vi "nanocal -- nuclear schottky fit V3.vi"() -> ()   [LabVIEW 2020] (continued)
\"κ0\"-> 0.000000001075  , \"mm1\"-> 0.000000000000  , \"mm2\"-> 0.000000000000  , \"mm3\"-> 0.000000000000  , \"T\"->  0.197000000000  , \"B\"-> 8.000000000000  , \"θ\"-> 90.000000000000  |>   , \r4103 ->   <| \"ζ\"->  0.162645417184  , \"τ1\"-> 0.023693851446  , \"τS\"-> 0.062400062170  , \"τN\"-> 0.026326088223  , \"τC\"-> 0.001322053294  , \"κ0\"-> 0.000000001070  , \"mm1\"-> 0.000000000000  , \"mm2\"-> 0.000000000000  , \"mm3\"-> 0.000000000000  , \"T\"->  0.197000000000  , \"B\"-> 7.000000000000  , \"θ\"-> 90.000000000000  |>   , \r4104 ->   <| \"ζ\"->  0.149904026692  , \"τ1\"-> 0.020347243982  , \"τS\"-> 0.075273674904  , \"τN\"-> 0.020640082408  , \"τC\"-> 0.001432916876  , \"κ0\"-> 0.000000001050  , \"mm1\"-> 0.000000000000  , \"mm2\"-> 0.000000000000  , \"mm3\"-> 0.000000000000  , \"T\"->  0.197000000000  , \"B\"-> 5.000000000000  , \"θ\"-> 90.000000000000  |>   , \r4105 ->   <| \"ζ\"->  0.121305227705  , \"τ1\"-> 0.032098202143  , \"τS\"-> 0.011865067519  , \"τN\"-> 0.005878702730  , \"τC\"-> 0.002147559783  , \"κ0\"-> 0.000000001032  , \"mm1\"-> 0.000000000000  , \"mm2\"-> 0.000000000000  , \"mm3\"-> 0.000000000000  , \"T\"->  0.197000000000  , \"B\"-> 0.000000000000  , \"θ\"-> 90.000000000000  |>   , \r4106 ->   <| \"ζ\"->  0.000000000000  , \"τ1\"-> 0.000000000000  , \"τS\"-> 0.000000000000  , \"τN\"-> 0.000000000000  , \"τC\"-> 0.000000000000  , \"κ0\"-> 0.000000000000  , \"mm1\"-> 0.000000000000  , \"mm2\"-> 0.000000000000  , \"mm3\"-> 0.000000000000  , \"T\"->  1.550000000000  , \"B\"-> 0.000000000000  , \"θ\"-> 90.000000000000  |>   , \r4107 ->   <| \"ζ\"->  0.000000000000  , \"τ1\"-> 0.000000000000  , \"τS\"-> 0.000000000000  , \"τN\"-> 0.000000000000  , \"τC\"-> 0.000000000000  , \"κ0\"-> 0.000000000000  , \"mm1\"-> 0.000000000000  , \"mm2\"-> 0.000000000000  , \"mm3\"-> 0.000000000000  , \"T\"->  1.000000000000  , \"B\"-> 0.000000000000  , \"θ\"-> 90.000000000000  |>   , \r4108 ->   <| \"ζ\"->  0.000000000000  , \"τ1\"-> 0.000000000000  , \"τS\"-> 0.000000000000  , \"τN\"-> 0.000000000000  , \"τC\"-> 0.000000000000  , \"κ0\"-> 0.000000000000  , \"mm1\"-> 0.000000000000  , \"mm2\"-> 0.000000000000  , \"mm3\"-> 0.000000000000  , \"T\"->  0.670000000000  , \"B\"-> 0.000000000000  , \"θ\"-> 90.000000000000  |>   , \r4110 ->   <| \"ζ\"->  0.282256587364  , \"τ1\"-> 0.041594214767  , \"τS\"-> 0.086147539104  , \"τN\"-> 0.179856853536  , \"τC\"-> 0.001095910669  , \"κ0\"-> 0.000000000648  , \"mm1\"-> 0.000000000000  , \"mm2\"-> 0.000000000000  , \"mm3\"-> 0.000000000000  , \"T\"->  0.160000000000  , \"B\"-> 12.000000000000  , \"θ\"-> 30.000000000000  |>   , \r4112 ->   <| \"ζ\"->  0.271363353906  , \"τ1\"-> 0.041443755069  , \"τS\"-> 0.099499603649  , \"τN\"-> 0.147006393002  , \"τC\"-> 0.001049141338  , \"κ0\"-> 0.000000000745  , \"mm1\"-> 0.000000000000  , \"mm2\"-> 0.000000000000  , \"mm3\"-> 0.000000000000  , \"T\"->  0.170000000000  , \"B\"-> 12.000000000000  , \"θ\"-> 30.000000000000  |>   , \r4113 ->   <| \"ζ\"->  0.338385515343  , \"τ1\"-> 0.049005471612  , \"τS\"-> 0.154718584573  , \"τN\"-> 0.405362096342  , \"τC\"-> 0.001218418583  , \"κ0\"-> 0.000000000425  , \"mm1\"-> 0.000000000000  , \"mm2\"-> 0.000000000000  , \"mm3\"-> 0.000000000000  , \"T\"->  0.140000000000  , \"B\"-> 12.000000000000  , \"θ\"-> 30.000000000000  |>   , \r4114 ->   <| \"ζ\"->  0.206936374087  , \"τ1\"-> 0.035561389628  , \"τS\"-> 0.073638069843  , \"τN\"-> 0.086460784567  , \"τC\"-> 0.001118747808  , \"κ0\"-> 0.000000001040  , \"mm1\"-> 0.000000000000  , \"mm2\"-> 0.000000000000  , \"mm3\"-> 0.000000000000  , \"T\"->  0.200000000000  , \"B\"-> 12.000000000000  , \"θ\"-> 30.000000000000  |>   , \r4115 ->   <| \"ζ\"->  0.117063376722  , \"τ1\"-> 0.028106174799  , \"τS\"-> 0.053754257200  , \"τN\"-> 0.028698663234  , \"τC\"-> 0.001316309287  , \"κ0\"-> 0.000000001351  , \"mm1\"-> 0.000000000000  , \"mm2\"-> 0.000000000000  , \"mm3\"-> 0.000000000000  , \"T\"->  0.250000000000  , \"B\"-> 12.000000000000  , \"θ\"-> 30.000000000000  |>   , \r4116 ->   <| \"ζ\"->  0.083503200365  , \"τ1\"-> 0.024154552454  , \"τS\"-> 0.043596505291  , \"τN\"-> 0.014415309061  , \"τC\"-> 0.001558050220  , \"κ0\"-> 0.000000001736  , \"mm1\"-> 0.000000000000  , \"mm2\"-> 0.000000000000  , \"mm3\"-> 0.000000000000  , \"T\"->  0.300000000000  , \"B\"-> 12.000000000000  , \"θ\"-> 30.000000000000  |>   , \r4117 ->   <| \"ζ\"->  0.066204854396  , \"τ1\"-> 0.022115453498  , \"τS\"-> 0.040315193272  , \"τN\"-> 0.009107814509  , \"τC\"-> 0.001932832854  , \"κ0\"-> 0.000000002123  , \"mm1\"-> 0.000000000000  , \"mm2\"-> 0.000000000000  , \"mm3\"-> 0.000000000000  , \"T\"->  0.360000000000  , \"B\"-> 12.000000000000  , \"θ\"-> 30.000000000000  |>   , \r4118 ->   <| \"ζ\"->  0.047151602613  , \"τ1\"-> 0.020449467018  , \"τS\"-> 0.034469980201  , \"τN\"-> 0.004383898226  , \"τC\"-> 0.002055617066  , \"κ0\"-> 0.000000002642  , \"mm1\"-> 0.000000000000  , \"mm2\"-> 0.000000000000  , \"mm3\"-> 0.000000000000  , \"T\"->  0.430000000000  , \"B\"-> 12.000000000000  , \"θ\"-> 30.000000000000  |>   , \r4119 ->   <| \"ζ\"->  0.034119623194  , \"τ1\"-> 0.019653386186  , \"τS\"-> 0.029887540037  , \"τN\"-> 0.002225158248  , \"τC\"-> 0.003041304002  , \"κ0\"-> 0.000000003299  , \"mm1\"-> 0.000000000000  , \"mm2\"-> 0.000000000000  , \"mm3\"-> 0.000000000000  , \"T\"->  0.530000000000  , \"B\"-> 12.000000000000  , \"θ\"-> 30.000000000000  |>   , \r4120 ->   <| \"ζ\"->  0.027646253689  , \"τ1\"-> 0.019846033328  , \"τS\"-> 0.026627790851  , \"τN\"-> 0.001396225568  , \"τC\"-> 0.003492513642  , \"κ0\"-> 0.000000003909  , \"mm1\"-> 0.000000000000  , \"mm2\"-> 0.000000000000  , \"mm3\"-> 0.000000000000  , \"T\"->  0.620000000000  , \"B\"-> 12.000000000000  , \"θ\"-> 30.000000000000  |>   , \r4121 ->   <| \"ζ\"->  0.021289486927  , \"τ1\"-> 0.020280543944  , \"τS\"-> 0.021209329853  , \"τN\"-> 0.000861491542  , \"τC\"-> 0.004079950225  , \"κ0\"-> 0.000000005431  , \"mm1\"-> 0.000000000000  , \"mm2\"-> 0.000000000000  , \"mm3\"-> 0.000000000000  , \"T\"->  0.830000000000  , \"B\"-> 12.000000000000  , \"θ\"-> 30.000000000000  |>   , \r4122 ->   <| \"ζ\"->  0.017438026946  , \"τ1\"-> 0.020462647610  , \"τS\"-> 0.016753258897  , \"τN\"-> 0.000520420479  , \"τC\"-> 0.004207921766  , \"κ0\"-> 0.000000007613  , \"mm1\"-> 0.000000000000  , \"mm2\"-> 0.000000000000  , \"mm3\"-> 0.000000000000  , \"T\"->  1.130000000000  , \"B\"-> 12.000000000000  , \"θ\"-> 30.000000000000  |>   , \r4123 ->   <| \"ζ\"->  0.016024491492  , \"τ1\"-> 0.020653048802  , \"τS\"-> 0.011065599363  , \"τN\"-> 0.000170904127  , \"τC\"-> 0.004501051440  , \"κ0\"-> 0.000000013123  , \"mm1\"-> 0.000000000000  , \"mm2\"-> 0.000000000000  , \"mm3\"-> 0.000000000000  , \"T\"->  1.900000000000  , \"B\"-> 12.000000000000  , \"θ\"-> 30.000000000000  |>   , \r4124 ->   <| \"ζ\"->  0.018571356814  , \"τ1\"-> 0.020537072361  , \"τS\"-> 0.007110096223  , \"τN\"-> 0.000081792866  , \"τC\"-> 0.004406299379  , \"κ0\"-> 0.000000023512  , \"mm1\"-> 0.000000000000  , \"mm2\"-> 0.000000000000  , \"mm3\"-> 0.000000000000  , \"T\"->  3.100000000000  , \"B\"-> 12.000000000000  , \"θ\"-> 30.000000000000  |>   , \r8026 ->   <| \"ζ\"->  0.226997000000  , \"τ1\"-> 0.061001000000  , \"τS\"-> 0.056065000000  , \"τN\"-> 0.451284000000  , \"τC\"-> 0.001917000000  , \"κ0\"-> 0.000000000541  , \"mm1\"-> 0.000000000000  , \"mm2\"-> 0.000000000000  , \"mm3\"-> 0.000000000000  , \"T\"->  0.127000000000  , \"B\"-> 12.000000000000  , \"θ\"-> 60.000000000000  |>   , \r8027 ->   <| \"ζ\"->  0.172926301574  , \"τ1\"-> 0.059570486348  , \"τS\"-> 0.050344582002  , \"τN\"-> 0.265837950917  , \"τC\"-> 0.001945823967  , \"κ0\"-> 0.000000000779  , \"mm1\"-> 0.000000000000  , \"mm2\"-> 0.000000000000  , \"mm3\"-> 0.000000000000  , \"T\"->  0.150000000000  , \"B\"-> 12.000000000000  , \"θ\"-> 60.000000000000  |>   , \r8028 ->   <| \"ζ\"->  0.148902664674  , \"τ1\"-> 0.053249092192  , \"τS\"-> 0.052262765310  , \"τN\"-> 0.169789454991  , \"τC\"-> 0.002259759037  , \"κ0\"-> 0.000000000876  , \"mm1\"-> 0.000000000000  , \"mm2\"-> 0.000000000000  , \"mm3\"-> 0.000000000000  , \"T\"->  0.179000000000  , \"B\"-> 12.000000000000  , \"θ\"-> 60.000000000000  |>   , \r8029 ->   <| \"ζ\"->  0.112487722964  , \"τ1\"-> 0.051395902330  , \"τS\"-> 0.046676654477  , \"τN\"-> 0.101658461283  , \"τC\"-> 0.002724334068  , \"κ0\"-> 0.000000001186  , \"mm1\"-> 0.000000000000  , \"mm2\"-> 0.000000000000  , \"mm3\"-> 0.000000000000  , \"T\"->  0.200000000000  , \"B\"-> 12.000000000000  , \"θ\"-> 60.000000000000  |>   , \r8030 ->   <| \"ζ\"->  0.086003233788  , \"τ1\"-> 0.048496801153  , \"τS\"-> 0.044168635092  , \"τN\"-> 0.056305790348  , \"τC\"-> 0.004231546790  , \"κ0\"-> 0.000000001462  , \"mm1\"-> 0.000000000000  , \"mm2\"-> 0.000000000000  , \"mm3\"-> 0.000000000000  , \"T\"->  0.240000000000  , \"B\"-> 12.000000000000  , \"θ\"-> 60.000000000000  |>   , \r8031 ->   <| \"ζ\"->  0.057384090127  , \"τ1\"-> 0.040985919910  , \"τS\"-> 0.035958032989  , \"τN\"-> 0.030082348419  , \"τC\"-> 0.004188092728  , \"κ0\"-> 0.000000001825  , \"mm1\"-> 0.000000000000  , \"mm2\"-> 0.000000000000  , \"mm3\"-> 0.000000000000  , \"T\"->  0.287000000000  , \"B\"-> 12.000000000000  , \"θ\"-> 60.000000000000  |>   , \r8032 ->   <| \"ζ\"->  0.043350504485  , \"τ1\"-> 0.035291986431  , \"τS\"-> 0.032748907144  , \"τN\"-> 0.017241468603  , \"τC\"-> 0.005241482788  , \"κ0\"-> 0.000000002152  , \"mm1\"-> 0.000000000000  , \"mm2\"-> 0.000000000000  , \"mm3\"-> 0.000000000000  , \"T\"->  0.330000000000  , \"B\"-> 12.000000000000  , \"θ\"-> 60.000000000000  |>   , \r8033 ->   <| \"ζ\"->  0.024739987039  , \"τ1\"-> 0.030389077736  , \"τS\"-> 0.031546934636  , \"τN\"-> 0.007979884290  , \"τC\"-> 0.005340402456  , \"κ0\"-> 0.000000002860  , \"mm1\"-> 0.000000000000  , \"mm2\"-> 0.000000000000  , \"mm3\"-> 0.000000000000  , \"T\"->  0.430000000000  , \"B\"-> 12.000000000000  , \"θ\"-> 60.000000000000  |>   , \r8034 ->   <| \"ζ\"->  0.017670248411  , \"τ1\"-> 0.029826184303  , \"τS\"-> 0.029273717282  , \"τN\"-> 0.004773699195  , \"τC\"-> 0.006202011547  , \"κ0\"-> 0.000000003450  , \"mm1\"-> 0.000000000000  , \"mm2\"-> 0.000000000000  , \"mm3\"-> 0.000000000000  , \"T\"->  0.510000000000  , \"B\"-> 12.000000000000  , \"θ\"-> 60.000000000000  |>   , \r8035 ->   <| \"ζ\"->  0.013857502217  , \"τ1\"-> 0.024739987039  , \"τS\"-> 0.022532031675  , \"τN\"-> 0.002673871537  , \"τC\"-> 0.006319058754  , \"κ0\"-> 0.000000004207  , \"mm1\"-> 0.000000000000  , \"mm2\"-> 0.000000000000  , \"mm3\"-> 0.000000000000  , \"T\"->  0.620000000000  , \"B\"-> 12.000000000000  , \"θ\"-> 60.000000000000  |>   , \r8036 ->   <| \"ζ\"->  0.008522550050  , \"τ1\"-> 0.024739987039  , \"τS\"-> 0.016706411949  , \"τN\"-> 0.001416010776  , \"τC\"-> 0.006938274982  , \"κ0\"-> 0.000000005839  , \"mm1\"-> 0.000000000000  , \"mm2\"-> 0.000000000000  , \"mm3\"-> 0.000000000000  , \"T\"->  0.830000000000  , \"B\"-> 12.000000000000  , \"θ\"-> 60.000000000000  |>   , \r8037 ->   <| \"ζ\"->  0.005755105359  , \"τ1\"-> 0.019922509440  , \"τS\"-> 0.014656977648  , \"τN\"-> 0.000670306824  , \"τC\"-> 0.007908429886  , \"κ0\"-> 0.000000008190  , \"mm1\"-> 0.000000000000  , \"mm2\"-> 0.000000000000  , \"mm3\"-> 0.000000000000  , \"T\"->  1.130000000000  , \"B\"-> 12.000000000000  , \"θ\"-> 60.000000000000  |>   , \r8038 ->   <| \"ζ\"->  0.003814320430  , \"τ1\"-> 0.018421720348  , \"τS\"-> 0.011291290594  , \"τN\"-> 0.000268276083  , \"τC\"-> 0.009845081970  , \"κ0\"-> 0.000000013900  , \"mm1\"-> 0.000000000000  , \"mm2\"-> 0.000000000000  , \"mm3\"-> 0.000000000000  , \"T\"->  1.900000000000  , \"B\"-> 12.000000000000  , \"θ\"-> 60.000000000000  |>   , \r8039 ->   <| \"ζ\"->  0.003101094202  , \"τ1\"-> 0.017947015305  , \"τS\"-> 0.009344228121  , \"τN\"-> 0.000104308237  , \"τC\"-> 0.008562742610  , \"κ0\"-> 0.000000024300  , \"mm1\"-> 0.000000000000  , \"mm2\"-> 0.000000000000  , \"mm3\"-> 0.000000000000  , \"T\"->  3.150000000000  , \"B\"-> 12.000000000000  , \"θ\"-> 60.000000000000  |>   , \r8040 ->   <| \"ζ\"->  0.002739426716  , \"τ1\"-> 0.017947015305  , \"τS\"-> 0.006831058554  , \"τN\"-> 0.000031540596  , \"τC\"-> 0.006316465842  , \"κ0\"-> 0.000000059000  , \"mm1\"-> 0.000000000000  , \"mm2\"-> 0.000000000000  , \"mm3\"-> 0.000000000000  , \"T\"->  5.700000000000  , \"B\"-> 12.000000000000  , \"θ\"-> 60.000000000000  |>   , \r8041 ->   <| \"ζ\"->  0.000000000000  , \"τ1\"-> 0.000000000000  , \"τS\"-> 0.000000000000  , \"τN\"-> 0.000000000000  , \"τC\"-> 0.000000000000  , \"κ0\"-> 0.000000000000  , \"mm1\"-> 0.000000000000  , \"mm2\"-> 0.000000000000  , \"mm3\"-> 0.000000000000  , \"T\"->  7.870000000000  , \"B\"-> 12.000000000000  , \"θ\"-> 60.000000000000  |>   , \r8042 ->   <| \"ζ\"->  0.000000000000  , \"τ1\"-> 0.000000000000  , \"τS\"-> 0.000000000000  , \"τN\"-> 0.000000000000  , \"τC\"-> 0.000000000000  , \"κ0\"-> 0.000000000000  , \"mm1\"-> 0.000000000000  , \"mm2\"-> 0.000000000000  , \"mm3\"-> 0.000000000000  , \"T\"->  9.800000000000  , \"B\"-> 12.000000000000  , \"θ\"-> 60.000000000000  |>   , \r8043 ->   <| \"ζ\"->  0.000000000000  , \"τ1\"-> 0.000000000000  , \"τS\"-> 0.000000000000  , \"τN\"-> 0.000000000000  , \"τC\"-> 0.000000000000  , \"κ0\"-> 0.000000000000  , \"mm1\"-> 0.000000000000  , \"mm2\"-> 0.000000000000  , \"mm3\"-> 0.000000000000  , \"T\"->  12.360000000000  , \"B\"-> 12.000000000000  , \"θ\"-> 60.000000000000  |>   , \r8044 ->   <| \"ζ\"->  0.000000000000  , \"τ1\"-> 0.000000000000  , \"τS\"-> 0.000000000000  , \"τN\"-> 0.000000000000  , \"τC\"-> 0.000000000000  , \"κ0\"-> 0.000000000000  , \"mm1\"-> 0.000000000000  , \"mm2\"-> 0.000000000000  , \"mm3\"-> 0.000000000000  , \"T\"->  14.800000000000  , \"B\"-> 12.000000000000  , \"θ\"-> 60.000000000000  |>   , \r8045 ->   <| \"ζ\"->  0.000000000000  , \"τ1\"-> 0.000000000000  , \"τS\"-> 0.000000000000  , \"τN\"-> 0.000000000000  , \"τC\"-> 0.000000000000  , \"κ0\"-> 0.000000000000  , \"mm1\"-> 0.000000000000  , \"mm2\"-> 0.000000000000  , \"mm3\"-> 0.000000000000  , \"T\"->  16.420000000000  , \"B\"-> 12.000000000000  , \"θ\"-> 60.000000000000  |>   , \r8046 ->   <| \"ζ\"->  0.000000000000  , \"τ1\"-> 0.000000000000  , \"τS\"-> 0.000000000000  , \"τN\"-> 0.000000000000  , \"τC\"-> 0.000000000000  , \"κ0\"-> 0.000000000000  , \"mm1\"-> 0.000000000000  , \"mm2\"-> 0.000000000000  , \"mm3\"-> 0.000000000000  , \"T\"->  18.040000000000  , \"B\"-> 12.000000000000  , \"θ\"-> 60.000000000000  |>   , \r8047 ->   <| \"ζ\"->  0.286336668596  , \"τ1\"-> 0.037477267671  , \"τS\"-> 0.354459287884  , \"τN\"-> 0.444916383639  , \"τC\"-> 0.001225600579  , \"κ0\"-> 0.000000000596  , \"mm1\"-> 0.000000000000  , \"mm2\"-> 0.000000000000  , \"mm3\"-> 0.000000000000  , \"T\"->  0.120000000000  , \"B\"-> 12.000000000000  , \"θ\"-> 0.000000000000  |>   , \r8048 ->   <| \"ζ\"->  0.219100303741  , \"τ1\"-> 0.028643012604  , \"τS\"-> 0.279362928811  , \"τN\"-> 0.246156444058  , \"τC\"-> 0.001272401549  , \"κ0\"-> 0.000000000760  , \"mm1\"-> 0.000000000000  , \"mm2\"-> 0.000000000000  , \"mm3\"-> 0.000000000000  , \"T\"->  0.148000000000  , \"B\"-> 12.000000000000  , \"θ\"-> 0.000000000000  |>   , \r8049 ->   <| \"ζ\"->  0.170488637524  , \"τ1\"-> 0.029234231120  , \"τS\"-> 0.149095458227  , \"τN\"-> 0.151792620275  , \"τC\"-> 0.001113424175  , \"κ0\"-> 0.000000001042  , \"mm1\"-> 0.000000000000  , \"mm2\"-> 0.000000000000  , \"mm3\"-> 0.000000000000  , \"T\"->  0.179000000000  , \"B\"-> 12.000000000000  , \"θ\"-> 0.000000000000  |>   , \r8050 ->   <| \"ζ\"->  0.130531197151  , \"τ1\"-> 0.025704482770  , \"τS\"-> 0.129606657196  , \"τN\"-> 0.091602369165  , \"τC\"-> 0.001441379995  , \"κ0\"-> 0.000000001211  , \"mm1\"-> 0.000000000000  , \"mm2\"-> 0.000000000000  , \"mm3\"-> 0.000000000000  , \"T\"->  0.197000000000  , \"B\"-> 12.000000000000  , \"θ\"-> 0.000000000000  |>   , \r8051 ->   <| \"ζ\"->  0.078258046754  , \"τ1\"-> 0.028009840731  , \"τS\"-> 0.092122038762  , \"τN\"-> 0.030129595899  , \"τC\"-> 0.001641062244  , \"κ0\"-> 0.000000001543  , \"mm1\"-> 0.000000000000  , \"mm2\"-> 0.000000000000  , \"mm3\"-> 0.000000000000  , \"T\"->  0.250000000000  , \"B\"-> 12.000000000000  , \"θ\"-> 0.000000000000  |>   , \r8052 ->   <| \"ζ\"->  0.054088186012  , \"τ1\"-> 0.023838802615  , \"τS\"-> 0.069079396629  , \"τN\"-> 0.016435267456  , \"τC\"-> 0.002025071743  , \"κ0\"-> 0.000000001955  , \"mm1\"-> 0.000000000000  , \"mm2\"-> 0.000000000000  , \"mm3\"-> 0.000000000000  , \"T\"->  0.300000000000  , \"B\"-> 12.000000000000  , \"θ\"-> 0.000000000000  |>   , \r8053 ->   <| \"ζ\"->  0.039314966212  , \"τ1\"-> 0.020712803909  , \"τS\"-> 0.055413767550  , \"τN\"-> 0.008474403424  , \"τC\"-> 0.002674063387  , \"κ0\"-> 0.000000002415  , \"mm1\"-> 0.000000000000  , \"mm2\"-> 0.000000000000  , \"mm3\"-> 0.000000000000  , \"T\"->  0.360000000000  , \"B\"-> 12.000000000000  , \"θ\"-> 0.000000000000  |>   , \r8054 ->   <| \"ζ\"->  0.031945976845  , \"τ1\"-> 0.019000922826  , \"τS\"-> 0.045624146388  , \"τN\"-> 0.005314716063  , \"τC\"-> 0.002488383471  , \"κ0\"-> 0.000000002954  , \"mm1\"-> 0.000000000000  , \"mm2\"-> 0.000000000000  , \"mm3\"-> 0.000000000000  , \"T\"->  0.430000000000  , \"B\"-> 12.000000000000  , \"θ\"-> 0.000000000000  |>   , \r8055 ->   <| \"ζ\"->  0.023031239946  , \"τ1\"-> 0.018268814012  , \"τS\"-> 0.037269400776  , \"τN\"-> 0.002696792890  , \"τC\"-> 0.003257395394  , \"κ0\"-> 0.000000003720  , \"mm1\"-> 0.000000000000  , \"mm2\"-> 0.000000000000  , \"mm3\"-> 0.000000000000  , \"T\"->  0.512000000000  , \"B\"-> 12.000000000000  , \"θ\"-> 0.000000000000  |>   , \r8056 ->   <| \"ζ\"->  0.019920170845  , \"τ1\"-> 0.016368892412  , \"τS\"-> 0.030579536580  , \"τN\"-> 0.001736017565  , \"τC\"-> 0.004971418152  , \"κ0\"-> 0.000000004410  , \"mm1\"-> 0.000000000000  , \"mm2\"-> 0.000000000000  , \"mm3\"-> 0.000000000000  , \"T\"->  0.610000000000  , \"B\"-> 12.000000000000  , \"θ\"-> 0.000000000000  |>   , \r8057 ->   <| \"ζ\"->  0.017558473054  , \"τ1\"-> 0.014545104284  , \"τS\"-> 0.022979681288  , \"τN\"-> 0.000840829385  , \"τC\"-> 0.005228030240  , \"κ0\"-> 0.000000006068  , \"mm1\"-> 0.000000000000  , \"mm2\"-> 0.000000000000  , \"mm3\"-> 0.000000000000  , \"T\"->  0.810000000000  , \"B\"-> 12.000000000000  , \"θ\"-> 0.000000000000  |>   , \r8058 ->   <| \"ζ\"->  0.011916480594  , \"τ1\"-> 0.012551282481  , \"τS\"-> 0.018233218660  , \"τN\"-> 0.000345702746  , \"τC\"-> 0.004699451527  , \"κ0\"-> 0.000000008451  , \"mm1\"-> 0.000000000000  , \"mm2\"-> 0.000000000000  , \"mm3\"-> 0.000000000000  , \"T\"->  1.120000000000  , \"B\"-> 12.000000000000  , \"θ\"-> 0.000000000000  |>   , \r8059 ->   <| \"ζ\"->  0.012831327568  , \"τ1\"-> 0.013315909415  , \"τS\"-> 0.012590836847  , \"τN\"-> 0.000065003013  , \"τC\"-> 0.005276356243  , \"κ0\"-> 0.000000013610  , \"mm1\"-> 0.000000000000  , \"mm2\"-> 0.000000000000  , \"mm3\"-> 0.000000000000  , \"T\"->  1.800000000000  , \"B\"-> 12.000000000000  , \"θ\"-> 0.000000000000  |>   , \r8060 ->   <| \"ζ\"->  0.019774146838  , \"τ1\"-> 0.013257273421  , \"τS\"-> 0.007064131508  , \"τN\"-> 0.000028000819  , \"τC\"-> 0.006942241845  , \"κ0\"-> 0.000000023477  , \"mm1\"-> 0.000000000000  , \"mm2\"-> 0.000000000000  , \"mm3\"-> 0.000000000000  , \"T\"->  3.000000000000  , \"B\"-> 12.000000000000  , \"θ\"-> 0.000000000000  |>   , \r8061 ->   <| \"ζ\"->  0.029251354442  , \"τ1\"-> 0.014634751206  , \"τS\"-> 0.003873958746  , \"τN\"-> 0.000007000487  , \"τC\"-> 0.006827504775  , \"κ0\"-> 0.000000056438  , \"mm1\"-> 0.000000000000  , \"mm2\"-> 0.000000000000  , \"mm3\"-> 0.000000000000  , \"T\"->  5.500000000000  , \"B\"-> 12.000000000000  , \"θ\"-> 0.000000000000  |>   , \r8070 ->   <| \"ζ\"->  0.161975781729  , \"τ1\"-> 0.073089805113  , \"τS\"-> 0.045018408115  , \"τN\"-> 0.161987434028  , \"τC\"-> 0.001482104484  , \"κ0\"-> 0.000000001038  , \"mm1\"-> 0.000000000000  , \"mm2\"-> 0.000000000000  , \"mm3\"-> 0.000000000000  , \"T\"->  0.179000000000  , \"B\"-> 12.000000000000  , \"θ\"-> 90.000000000000  |>   , \r8071 ->   <| \"ζ\"->  0.300863384227  , \"τ1\"-> 0.104924004009  , \"τS\"-> 0.071070599729  , \"τN\"-> 0.992887187112  , \"τC\"-> 0.001721587800  , \"κ0\"-> 0.000000000548  , \"mm1\"-> 0.000000000000  , \"mm2\"-> 0.000000000000  , \"mm3\"-> 0.000000000000  , \"T\"->  0.120000000000  , \"B\"-> 12.000000000000  , \"θ\"-> 90.000000000000  |>   , \r8072 ->   <| \"ζ\"->  0.215697702358  , \"τ1\"-> 0.095971807771  , \"τS\"-> 0.069319630290  , \"τN\"-> 0.366712218878  , \"τC\"-> 0.001526252261  , \"κ0\"-> 0.000000000784  , \"mm1\"-> 0.000000000000  , \"mm2\"-> 0.000000000000  , \"mm3\"-> 0.000000000000  , \"T\"->  0.148000000000  , \"B\"-> 12.000000000000  , \"θ\"-> 90.000000000000  |>   , \r8073 ->   <| \"ζ\"->  0.139117463690  , \"τ1\"-> 0.070330410174  , \"τS\"-> 0.040829719954  , \"τN\"-> 0.122434321115  , \"τC\"-> 0.001436112939  , \"κ0\"-> 0.000000001208  , \"mm1\"-> 0.000000000000  , \"mm2\"-> 0.000000000000  , \"mm3\"-> 0.000000000000  , \"T\"->  0.197000000000  , \"B\"-> 12.000000000000  , \"θ\"-> 90.000000000000  |>   , \r8074 ->   <| \"ζ\"->  0.079912790251  , \"τ1\"-> 0.053932962768  , \"τS\"-> 0.033847624645  , \"τN\"-> 0.047947649984  , \"τC\"-> 0.001828917906  , \"κ0\"-> 0.000000001546  , \"mm1\"-> 0.000000000000  , \"mm2\"-> 0.000000000000  , \"mm3\"-> 0.000000000000  , \"T\"->  0.249000000000  , \"B\"-> 12.000000000000  , \"θ\"-> 90.000000000000  |>   , \r8075 ->   <| \"ζ\"->  0.057938569833  , \"τ1\"-> 0.045244527663  , \"τS\"-> 0.029709028064  , \"τN\"-> 0.023577376257  , \"τC\"-> 0.002006607539  , \"κ0\"-> 0.000000001948  , \"mm1\"-> 0.000000000000  , \"mm2\"-> 0.000000000000  , \"mm3\"-> 0.000000000000  , \"T\"->  0.300000000000  , \"B\"-> 12.000000000000  , \"θ\"-> 90.000000000000  |>   , \r8076 ->   <| \"ζ\"->  0.044154556051  , \"τ1\"-> 0.038823125235  , \"τS\"-> 0.027069314930  , \"τN\"-> 0.013601990730  , \"τC\"-> 0.002287979276  , \"κ0\"-> 0.000000002359  , \"mm1\"-> 0.000000000000  , \"mm2\"-> 0.000000000000  , \"mm3\"-> 0.000000000000  , \"T\"->  0.360000000000  , \"B\"-> 12.000000000000  , \"θ\"-> 90.000000000000  |>   , \r8077 ->   <| \"ζ\"->  0.032748569996  , \"τ1\"-> 0.031072007290  , \"τS\"-> 0.024343937548  , \"τN\"-> 0.006961654481  , \"τC\"-> 0.002967111565  , \"κ0\"-> 0.000000002964  , \"mm1\"-> 0.000000000000  , \"mm2\"-> 0.000000000000  , \"mm3\"-> 0.000000000000  , \"T\"->  0.430000000000  , \"B\"-> 12.000000000000  , \"θ\"-> 90.000000000000  |>   , \r8078 ->   <| \"ζ\"->  0.027599263457  , \"τ1\"-> 0.026239105728  , \"τS\"-> 0.022370859308  , \"τN\"-> 0.003857632966  , \"τC\"-> 0.003499360499  , \"κ0\"-> 0.000000003681  , \"mm1\"-> 0.000000000000  , \"mm2\"-> 0.000000000000  , \"mm3\"-> 0.000000000000  , \"T\"->  0.512000000000  , \"B\"-> 12.000000000000  , \"θ\"-> 90.000000000000  |>   , \r8079 ->   <| \"ζ\"->  0.020568815513  , \"τ1\"-> 0.023045965648  , \"τS\"-> 0.020791387386  , \"τN\"-> 0.002229171297  , \"τC\"-> 0.004427475438  , \"κ0\"-> 0.000000004398  , \"mm1\"-> 0.000000000000  , \"mm2\"-> 0.000000000000  , \"mm3\"-> 0.000000000000  , \"T\"->  0.610000000000  , \"B\"-> 12.000000000000  , \"θ\"-> 90.000000000000  |>   , \r8080 ->   <| \"ζ\"->  0.016548170999  , \"τ1\"-> 0.020108887890  , \"τS\"-> 0.018558394948  , \"τN\"-> 0.001160732495  , \"τC\"-> 0.004746126241  , \"κ0\"-> 0.000000005882  , \"mm1\"-> 0.000000000000  , \"mm2\"-> 0.000000000000  , \"mm3\"-> 0.000000000000  , \"T\"->  0.810000000000  , \"B\"-> 12.000000000000  , \"θ\"-> 90.000000000000  |>   , \r8081 ->   <| \"ζ\"->  0.014495870556  , \"τ1\"-> 0.019990087457  , \"τS\"-> 0.016832201384  , \"τN\"-> 0.000455517238  , \"τC\"-> 0.005555782498  , \"κ0\"-> 0.000000008420  , \"mm1\"-> 0.000000000000  , \"mm2\"-> 0.000000000000  , \"mm3\"-> 0.000000000000  , \"T\"->  1.100000000000  , \"B\"-> 12.000000000000  , \"θ\"-> 90.000000000000  |>   , \r8082 ->   <| \"ζ\"->  0.014043763709  , \"τ1\"-> 0.018292068543  , \"τS\"-> 0.011311396743  , \"τN\"-> 0.000128802259  , \"τC\"-> 0.008087849636  , \"κ0\"-> 0.000000014258  , \"mm1\"-> 0.000000000000  , \"mm2\"-> 0.000000000000  , \"mm3\"-> 0.000000000000  , \"T\"->  1.800000000000  , \"B\"-> 12.000000000000  , \"θ\"-> 90.000000000000  |>   , \r8083 ->   <| \"ζ\"->  0.016187684631  , \"τ1\"-> 0.018325345271  , \"τS\"-> 0.007510087776  , \"τN\"-> 0.000028419157  , \"τC\"-> 0.008115463080  , \"κ0\"-> 0.000000024747  , \"mm1\"-> 0.000000000000  , \"mm2\"-> 0.000000000000  , \"mm3\"-> 0.000000000000  , \"T\"->  3.000000000000  , \"B\"-> 12.000000000000  , \"θ\"-> 90.000000000000  |>   , \r8084 ->   <| \"ζ\"->  0.027897403691  , \"τ1\"-> 0.014639690770  , \"τS\"-> 0.004105291179  , \"τN\"-> 0.000006999171  , \"τC\"-> 0.007414449545  , \"κ0\"-> 0.000000059701  , \"mm1\"-> 0.000000000000  , \"mm2\"-> 0.000000000000  , \"mm3\"-> 0.000000000000  , \"T\"->  5.700000000000  , \"B\"-> 12.000000000000  , \"θ\"-> 90.000000000000  |>   , \r8094 ->   <| \"ζ\"->  0.000000000000  , \"τ1\"-> 0.000000000000  , \"τS\"-> 0.000000000000  , \"τN\"-> 0.000000000000  , \"τC\"-> 0.000000000000  , \"κ0\"-> 0.000000000000  , \"mm1\"-> 0.000000000000  , \"mm2\"-> 0.000000000000  , \"mm3\"-> 0.000000000000  , \"T\"->  0.300000000000  , \"B\"-> 6.000000000000  , \"θ\"-> 90.000000000000  |>   , \r8095 ->   <| \"ζ\"->  0.132901556203  , \"τ1\"-> 0.022795175616  , \"τS\"-> 0.082481385864  , \"τN\"-> 0.041432545456  , \"τC\"-> 0.001408424074  , \"κ0\"-> 0.000000001182  , \"mm1\"-> 0.000000000000  , \"mm2\"-> 0.000000000000  , \"mm3\"-> 0.000000000000  , \"T\"->  0.197000000000  , \"B\"-> 6.000000000000  , \"θ\"-> 90.000000000000  |>   , \r8098 ->   <| \"ζ\"->  0.000000000000  , \"τ1\"-> 0.000000000000  , \"τS\"-> 0.000000000000  , \"τN\"-> 0.000000000000  , \"τC\"-> 0.000000000000  , \"κ0\"-> 0.000000000000  , \"mm1\"-> 0.000000000000  , \"mm2\"-> 0.000000000000  , \"mm3\"-> 0.000000000000  , \"T\"->  0.148000000000  , \"B\"-> 6.000000000000  , \"θ\"-> 90.000000000000  |>   , \r8099 ->   <| \"ζ\"->  0.132534999612  , \"τ1\"-> 0.042581417401  , \"τS\"-> 0.054103824371  , \"τN\"-> 0.072163013930  , \"τC\"-> 0.001421040158  , \"κ0\"-> 0.000000001190  , \"mm1\"-> 0.000000000000  , \"mm2\"-> 0.000000000000  , \"mm3\"-> 0.000000000000  , \"T\"->  0.197000000000  , \"B\"-> 9.000000000000  , \"θ\"-> 90.000000000000  |>   , \r8100 ->   <| \"ζ\"->  0.124414912597  , \"τ1\"-> 0.052685716706  , \"τS\"-> 0.041788480794  , \"τN\"-> 0.092820346766  , \"τC\"-> 0.001183564004  , \"κ0\"-> 0.000000001217  , \"mm1\"-> 0.000000000000  , \"mm2\"-> 0.000000000000  , \"mm3\"-> 0.000000000000  , \"T\"->  0.197000000000  , \"B\"-> 11.000000000000  , \"θ\"-> 90.000000000000  |>   , \r8101 ->   <| \"ζ\"->  0.130083148284  , \"τ1\"-> 0.046211117525  , \"τS\"-> 0.046173592526  , \"τN\"-> 0.081942172735  , \"τC\"-> 0.001380184863  , \"κ0\"-> 0.000000001209  , \"mm1\"-> 0.000000000000  , \"mm2\"-> 0.000000000000  , \"mm3\"-> 0.000000000000  , \"T\"->  0.197000000000  , \"B\"-> 10.000000000000  , \"θ\"-> 90.000000000000  |>   , \r8102 ->   <| \"ζ\"->  0.126440702434  , \"τ1\"-> 0.034118036572  , \"τS\"-> 0.060921114440  , \"τN\"-> 0.059832148427  , \"τC\"-> 0.001404471084  , \"κ0\"-> 0.000000001199  , \"mm1\"-> 0.000000000000  , \"mm2\"-> 0.000000000000  , \"mm3\"-> 0.000000000000  , \"T\"->  0.197000000000  , \"B\"-> 8.000000000000  , \"θ\"-> 90.000000000000  |>   , \r8103 ->   <| \"ζ\"->  0.131383255045  , \"τ1\"-> 0.026827335842  , \"τS\"-> 0.071725959535  , \"τN\"-> 0.047510049318  , \"τC\"-> 0.001407613780  , \"κ0\"-> 0.000000001187  , \"mm1\"-> 0.000000000000  , \"mm2\"-> 0.000000000000  , \"mm3\"-> 0.000000000000  , \"T\"->  0.197000000000  , \"B\"-> 7.000000000000  , \"θ\"-> 90.000000000000  |>   , \r8104 ->   <| \"ζ\"->  0.125455081262  , \"τ1\"-> 0.021777951907  , \"τS\"-> 0.089086097551  , \"τN\"-> 0.033580911935  , \"τC\"-> 0.001437991682  , \"κ0\"-> 0.000000001167  , \"mm1\"-> 0.000000000000  , \"mm2\"-> 0.000000000000  , \"mm3\"-> 0.000000000000  , \"T\"->  0.197000000000  , \"B\"-> 5.000000000000  , \"θ\"-> 90.000000000000  |>   , \r8105 ->   <| \"ζ\"->  0.101804363109  , \"τ1\"-> 0.031947692776  , \"τS\"-> 0.014125667853  , \"τN\"-> 0.006009042128  , \"τC\"-> 0.002323789932  , \"κ0\"-> 0.000000001168  , \"mm1\"-> 0.000000000000  , \"mm2\"-> 0.000000000000  , \"mm3\"-> 0.000000000000  , \"T\"->  0.197000000000  , \"B\"-> 0.000000000000  , \"θ\"-> 90.000000000000  |>   , \r8106 ->   <| \"ζ\"->  0.000000000000  , \"τ1\"-> 0.000000000000  , \"τS\"-> 0.000000000000  , \"τN\"-> 0.000000000000  , \"τC\"-> 0.000000000000  , \"κ0\"-> 0.000000000000  , \"mm1\"-> 0.000000000000  , \"mm2\"-> 0.000000000000  , \"mm3\"-> 0.000000000000  , \"T\"->  1.550000000000  , \"B\"-> 0.000000000000  , \"θ\"-> 90.000000000000  |>   , \r8107 ->   <| \"ζ\"->  0.000000000000  , \"τ1\"-> 0.000000000000  , \"τS\"-> 0.000000000000  , \"τN\"-> 0.000000000000  , \"τC\"-> 0.000000000000  , \"κ0\"-> 0.000000000000  , \"mm1\"-> 0.000000000000  , \"mm2\"-> 0.000000000000  , \"mm3\"-> 0.000000000000  , \"T\"->  1.000000000000  , \"B\"-> 0.000000000000  , \"θ\"-> 90.000000000000  |>   , \r8108 ->   <| \"ζ\"->  0.000000000000  , \"τ1\"-> 0.000000000000  , \"τS\"-> 0.000000000000  , \"τN\"-> 0.000000000000  , \"τC\"-> 0.000000000000  , \"κ0\"-> 0.000000000000  , \"mm1\"-> 0.000000000000  , \"mm2\"-> 0.000000000000  , \"mm3\"-> 0.000000000000  , \"T\"->  0.670000000000  , \"B\"-> 0.000000000000  , \"θ\"-> 90.000000000000  |>   , \r8110 ->   <| \"ζ\"->  0.162585495535  , \"τ1\"-> 0.037883389730  , \"τS\"-> 0.086562863191  , \"τN\"-> 0.241872534356  , \"τC\"-> 0.001506143871  , \"κ0\"-> 0.000000000791  , \"mm1\"-> 0.000000000000  , \"mm2\"-> 0.000000000000  , \"mm3\"-> 0.000000000000  , \"T\"->  0.160000000000  , \"B\"-> 12.000000000000  , \"θ\"-> 30.000000000000  |>   , \r8112 ->   <| \"ζ\"->  0.156472219566  , \"τ1\"-> 0.031017925061  , \"τS\"-> 0.080872234530  , \"τN\"-> 0.219381306397  , \"τC\"-> 0.001437792153  , \"κ0\"-> 0.000000000867  , \"mm1\"-> 0.000000000000  , \"mm2\"-> 0.000000000000  , \"mm3\"-> 0.000000000000  , \"T\"->  0.170000000000  , \"B\"-> 12.000000000000  , \"θ\"-> 30.000000000000  |>   , \r8113 ->   <| \"ζ\"->  0.211545693132  , \"τ1\"-> 0.029106147473  , \"τS\"-> 0.094475691604  , \"τN\"-> 0.369151052631  , \"τC\"-> 0.001396700790  , \"κ0\"-> 0.000000000537  , \"mm1\"-> 0.000000000000  , \"mm2\"-> 0.000000000000  , \"mm3\"-> 0.000000000000  , \"T\"->  0.140000000000  , \"B\"-> 12.000000000000  , \"θ\"-> 30.000000000000  |>   , \r8114 ->   <| \"ζ\"->  0.128615765969  , \"τ1\"-> 0.032665502211  , \"τS\"-> 0.082694869013  , \"τN\"-> 0.105788373632  , \"τC\"-> 0.001439686784  , \"κ0\"-> 0.000000001168  , \"mm1\"-> 0.000000000000  , \"mm2\"-> 0.000000000000  , \"mm3\"-> 0.000000000000  , \"T\"->  0.200000000000  , \"B\"-> 12.000000000000  , \"θ\"-> 30.000000000000  |>   , \r8115 ->   <| \"ζ\"->  0.072634365939  , \"τ1\"-> 0.028637109000  , \"τS\"-> 0.065061142288  , \"τN\"-> 0.040304243071  , \"τC\"-> 0.001622979999  , \"κ0\"-> 0.000000001498  , \"mm1\"-> 0.000000000000  , \"mm2\"-> 0.000000000000  , \"mm3\"-> 0.000000000000  , \"T\"->  0.250000000000  , \"B\"-> 12.000000000000  , \"θ\"-> 30.000000000000  |>   , \r8116 ->   <| \"ζ\"->  0.050663808076  , \"τ1\"-> 0.024940898568  , \"τS\"-> 0.056803871413  , \"τN\"-> 0.018856862265  , \"τC\"-> 0.002133501904  , \"κ0\"-> 0.000000001888  , \"mm1\"-> 0.000000000000  , \"mm2\"-> 0.000000000000  , \"mm3\"-> 0.000000000000  , \"T\"->  0.300000000000  , \"B\"-> 12.000000000000  , \"θ\"-> 30.000000000000  |>   , \r8117 ->   <| \"ζ\"->  0.036420486357  , \"τ1\"-> 0.020986681106  , \"τS\"-> 0.049149577509  , \"τN\"-> 0.011109585503  , \"τC\"-> 0.002819780093  , \"κ0\"-> 0.000000002299  , \"mm1\"-> 0.000000000000  , \"mm2\"-> 0.000000000000  , \"mm3\"-> 0.000000000000  , \"T\"->  0.360000000000  , \"B\"-> 12.000000000000  , \"θ\"-> 30.000000000000  |>   , \r8118 ->   <| \"ζ\"->  0.028468689077  , \"τ1\"-> 0.020220821810  , \"τS\"-> 0.043529484347  , \"τN\"-> 0.005653540941  , \"τC\"-> 0.003150537442  , \"κ0\"-> 0.000000002855  , \"mm1\"-> 0.000000000000  , \"mm2\"-> 0.000000000000  , \"mm3\"-> 0.000000000000  , \"T\"->  0.430000000000  , \"B\"-> 12.000000000000  , \"θ\"-> 30.000000000000  |>   , \r8119 ->   <| \"ζ\"->  0.021116250068  , \"τ1\"-> 0.020669239851  , \"τS\"-> 0.037941648749  , \"τN\"-> 0.003221866945  , \"τC\"-> 0.003619427775  , \"κ0\"-> 0.000000003553  , \"mm1\"-> 0.000000000000  , \"mm2\"-> 0.000000000000  , \"mm3\"-> 0.000000000000  , \"T\"->  0.530000000000  , \"B\"-> 12.000000000000  , \"θ\"-> 30.000000000000  |>   , \r8120 ->   <| \"ζ\"->  0.016892016292  , \"τ1\"-> 0.020344757415  , \"τS\"-> 0.033845756966  , \"τN\"-> 0.001946817417  , \"τC\"-> 0.004013762913  , \"κ0\"-> 0.000000004252  , \"mm1\"-> 0.000000000000  , \"mm2\"-> 0.000000000000  , \"mm3\"-> 0.000000000000  , \"T\"->  0.620000000000  , \"B\"-> 12.000000000000  , \"θ\"-> 30.000000000000  |>   , \r8121 ->   <| \"ζ\"->  0.013460153434  , \"τ1\"-> 0.020684726260  , \"τS\"-> 0.027140346721  , \"τN\"-> 0.000960302406  , \"τC\"-> 0.004517434882  , \"κ0\"-> 0.000000005889  , \"mm1\"-> 0.000000000000  , \"mm2\"-> 0.000000000000  , \"mm3\"-> 0.000000000000  , \"T\"->  0.830000000000  , \"B\"-> 12.000000000000  , \"θ\"-> 30.000000000000  |>   , \r8122 ->   <| \"ζ\"->  0.010912011148  , \"τ1\"-> 0.020760977312  , \"τS\"-> 0.021106239637  , \"τN\"-> 0.000452316988  , \"τC\"-> 0.005003723454  , \"κ0\"-> 0.000000008194  , \"mm1\"-> 0.000000000000  , \"mm2\"-> 0.000000000000  , \"mm3\"-> 0.000000000000  , \"T\"->  1.130000000000  , \"B\"-> 12.000000000000  , \"θ\"-> 30.000000000000  |>   , \r8123 ->   <| \"ζ\"->  0.009772435939  , \"τ1\"-> 0.020827345370  , \"τS\"-> 0.013809334085  , \"τN\"-> 0.000168485133  , \"τC\"-> 0.005555066716  , \"κ0\"-> 0.000000013930  , \"mm1\"-> 0.000000000000  , \"mm2\"-> 0.000000000000  , \"mm3\"-> 0.000000000000  , \"T\"->  1.900000000000  , \"B\"-> 12.000000000000  , \"θ\"-> 30.000000000000  |>   , \r8124 ->   <| \"ζ\"->  0.010111127240  , \"τ1\"-> 0.020788755574  , \"τS\"-> 0.009968978424  , \"τN\"-> 0.000077788811  , \"τC\"-> 0.004598584548  , \"κ0\"-> 0.000000024346  , \"mm1\"-> 0.000000000000  , \"mm2\"-> 0.000000000000  , \"mm3\"-> 0.000000000000  , \"T\"->  3.100000000000  , \"B\"-> 12.000000000000  , \"θ\"-> 30.000000000000  |>   , \r40047 ->   <| \"ζ\"->  0.020744689680  , \"τ1\"-> 0.017944253087  , \"τS\"-> 0.003548154619  , \"τN\"-> 0.000036329906  , \"τC\"-> 0.004738266852  , \"κ0\"-> 0.000000058027  , \"mm1\"-> 0.000000000000  , \"mm2\"-> 0.000000000000  , \"mm3\"-> 0.000000000000  , \"T\"->  19.600000000000  , \"B\"-> 12.000000000000  , \"θ\"-> 60.000000000000  |>   , \r40049 ->   <| \"ζ\"->  0.334519022578  , \"τ1\"-> 0.071617660141  , \"τS\"-> 0.066230384072  , \"τN\"-> 0.374518999658  , \"τC\"-> 0.002158821958  , \"κ0\"-> 0.000000000405  , \"mm1\"-> 0.000000000000  , \"mm2\"-> 0.000000000000  , \"mm3\"-> 0.000000000000  , \"T\"->  0.129000000000  , \"B\"-> 12.000000000000  , \"θ\"-> 60.000000000000  |>   , \r40125 ->   <| \"ζ\"->  0.295520923520  , \"τ1\"-> 0.054772440405  , \"τS\"-> 0.071814005451  , \"τN\"-> 0.249593767169  , \"τC\"-> 0.001103632155  , \"κ0\"-> 0.000000000625  , \"mm1\"-> 0.000000000000  , \"mm2\"-> 0.000000000000  , \"mm3\"-> 0.000000000000  , \"T\"->  0.157000000000  , \"B\"-> 12.000000000000  , \"θ\"-> 45.000000000000  |>   , \r40126 ->   <| \"ζ\"->  0.523545279740  , \"τ1\"-> 0.065613539167  , \"τS\"-> 0.100000000000  , \"τN\"-> 0.424083114177  , \"τC\"-> 0.000911255863  , \"κ0\"-> 0.000000000418  , \"mm1\"-> 0.000000000000  , \"mm2\"-> 0.000000000000  , \"mm3\"-> 0.000000000000  , \"T\"->  0.120000000000  , \"B\"-> 12.000000000000  , \"θ\"-> 45.000000000000  |>   , \r40127 ->   <| \"ζ\"->  0.273742116471  , \"τ1\"-> 0.052262909995  , \"τS\"-> 0.060554036646  , \"τN\"-> 0.154269705680  , \"τC\"-> 0.001074144337  , \"κ0\"-> 0.000000000753  , \"mm1\"-> 0.000000000000  , \"mm2\"-> 0.000000000000  , \"mm3\"-> 0.000000000000  , \"T\"->  0.170000000000  , \"B\"-> 12.000000000000  , \"θ\"-> 45.000000000000  |>   , \r40128 ->   <| \"ζ\"->  0.215688135788  , \"τ1\"-> 0.043710888546  , \"τS\"-> 0.044756474141  , \"τN\"-> 0.090222547904  , \"τC\"-> 0.001049781785  , \"κ0\"-> 0.000000001047  , \"mm1\"-> 0.000000000000  , \"mm2\"-> 0.000000000000  , \"mm3\"-> 0.000000000000  , \"T\"->  0.200000000000  , \"B\"-> 12.000000000000  , \"θ\"-> 45.000000000000  |>   , \r40129 ->   <| \"ζ\"->  0.118583992968  , \"τ1\"-> 0.035232851003  , \"τS\"-> 0.037458022816  , \"τN\"-> 0.033724509363  , \"τC\"-> 0.001440922263  , \"κ0\"-> 0.000000001360  , \"mm1\"-> 0.000000000000  , \"mm2\"-> 0.000000000000  , \"mm3\"-> 0.000000000000  , \"T\"->  0.255000000000  , \"B\"-> 12.000000000000  , \"θ\"-> 45.000000000000  |>   , \r40130 ->   <| \"ζ\"->  0.085152769414  , \"τ1\"-> 0.029001116263  , \"τS\"-> 0.032604663993  , \"τN\"-> 0.016878763935  , \"τC\"-> 0.001443524845  , \"κ0\"-> 0.000000001728  , \"mm1\"-> 0.000000000000  , \"mm2\"-> 0.000000000000  , \"mm3\"-> 0.000000000000  , \"T\"->  0.300000000000  , \"B\"-> 12.000000000000  , \"θ\"-> 45.000000000000  |>   , \r40131 ->   <| \"ζ\"->  0.061011838044  , \"τ1\"-> 0.025440548989  , \"τS\"-> 0.030028053978  , \"τN\"-> 0.010140731955  , \"τC\"-> 0.001895079687  , \"κ0\"-> 0.000000002115  , \"mm1\"-> 0.000000000000  , \"mm2\"-> 0.000000000000  , \"mm3\"-> 0.000000000000  , \"T\"->  0.360000000000  , \"B\"-> 12.000000000000  , \"θ\"-> 45.000000000000  |>   , \r40132 ->   <| \"ζ\"->  0.046686299518  , \"τ1\"-> 0.021011215626  , \"τS\"-> 0.027633142317  , \"τN\"-> 0.005348477555  , \"τC\"-> 0.002098477650  , \"κ0\"-> 0.000000002635  , \"mm1\"-> 0.000000000000  , \"mm2\"-> 0.000000000000  , \"mm3\"-> 0.000000000000  , \"T\"->  0.430000000000  , \"B\"-> 12.000000000000  , \"θ\"-> 45.000000000000  |>   , \r40133 ->   <| \"ζ\"->  0.035204330012  , \"τ1\"-> 0.021011523093  , \"τS\"-> 0.025247316079  , \"τN\"-> 0.002718647875  , \"τC\"-> 0.003091727575  , \"κ0\"-> 0.000000003296  , \"mm1\"-> 0.000000000000  , \"mm2\"-> 0.000000000000  , \"mm3\"-> 0.000000000000  , \"T\"->  0.530000000000  , \"B\"-> 12.000000000000  , \"θ\"-> 45.000000000000  |>   , \r40134 ->   <| \"ζ\"->  0.030862035723  , \"τ1\"-> 0.019328530751  , \"τS\"-> 0.023568572597  , \"τN\"-> 0.001701966614  , \"τC\"-> 0.003453790534  , \"κ0\"-> 0.000000003906  , \"mm1\"-> 0.000000000000  , \"mm2\"-> 0.000000000000  , \"mm3\"-> 0.000000000000  , \"T\"->  0.620000000000  , \"B\"-> 12.000000000000  , \"θ\"-> 45.000000000000  |>   , \r40135 ->   <| \"ζ\"->  0.023591124045  , \"τ1\"-> 0.014910006225  , \"τS\"-> 0.019342950404  , \"τN\"-> 0.000752972387  , \"τC\"-> 0.004900413232  , \"κ0\"-> 0.000000005453  , \"mm1\"-> 0.000000000000  , \"mm2\"-> 0.000000000000  , \"mm3\"-> 0.000000000000  , \"T\"->  0.830000000000  , \"B\"-> 12.000000000000  , \"θ\"-> 45.000000000000  |>   , \r40136 ->   <| \"ζ\"->  0.020215154826  , \"τ1\"-> 0.014105227254  , \"τS\"-> 0.015660924043  , \"τN\"-> 0.000525137036  , \"τC\"-> 0.005447728357  , \"κ0\"-> 0.000000007594  , \"mm1\"-> 0.000000000000  , \"mm2\"-> 0.000000000000  , \"mm3\"-> 0.000000000000  , \"T\"->  1.130000000000  , \"B\"-> 12.000000000000  , \"θ\"-> 45.000000000000  |>   , \r40137 ->   <| \"ζ\"->  0.018090572724  , \"τ1\"-> 0.013314780956  , \"τS\"-> 0.010820835010  , \"τN\"-> 0.000265552167  , \"τC\"-> 0.005393540417  , \"κ0\"-> 0.000000013100  , \"mm1\"-> 0.000000000000  , \"mm2\"-> 0.000000000000  , \"mm3\"-> 0.000000000000  , \"T\"->  1.900000000000  , \"B\"-> 12.000000000000  , \"θ\"-> 45.000000000000  |>   , \r40138 ->   <| \"ζ\"->  0.019438138135  , \"τ1\"-> 0.013521019406  , \"τS\"-> 0.007253169401  , \"τN\"-> 0.000154824830  , \"τC\"-> 0.004746579385  , \"κ0\"-> 0.000000023466  , \"mm1\"-> 0.000000000000  , \"mm2\"-> 0.000000000000  , \"mm3\"-> 0.000000000000  , \"T\"->  3.100000000000  , \"B\"-> 12.000000000000  , \"θ\"-> 45.000000000000  |>   , \r40139 ->   <| \"ζ\"->  0.018573189054  , \"τ1\"-> 0.013304612245  , \"τS\"-> 0.003723860844  , \"τN\"-> 0.000084829442  , \"τC\"-> 0.004309703632  , \"κ0\"-> 0.000000058362  , \"mm1\"-> 0.000000000000  , \"mm2\"-> 0.000000000000  , \"mm3\"-> 0.000000000000  , \"T\"->  5.700000000000  , \"B\"-> 12.000000000000  , \"θ\"-> 45.000000000000  |>   , \r80047 ->   <| \"ζ\"->  0.000000000000  , \"τ1\"-> 0.000000000000  , \"τS\"-> 0.000000000000  , \"τN\"-> 0.000000000000  , \"τC\"-> 0.000000000000  , \"κ0\"-> 0.000000000000  , \"mm1\"-> 0.000000000000  , \"mm2\"-> 0.000000000000  , \"mm3\"-> 0.000000000000  , \"T\"->  19.600000000000  , \"B\"-> 12.000000000000  , \"θ\"-> 60.000000000000  |>   , \r80049 ->   <| \"ζ\"->  0.206128000000  , \"τ1\"-> 0.061001000000  , \"τS\"-> 0.056065000000  , \"τN\"-> 0.442324169403  , \"τC\"-> 0.001917000000  , \"κ0\"-> 0.000000000541  , \"mm1\"-> 0.000000000000  , \"mm2\"-> 0.000000000000  , \"mm3\"-> 0.000000000000  , \"T\"->  0.129000000000  , \"B\"-> 12.000000000000  , \"θ\"-> 60.000000000000  |>   , \r80125 ->   <| \"ζ\"->  0.000000000000  , \"τ1\"-> 0.000000000000  , \"τS\"-> 0.000000000000  , \"τN\"-> 0.000000000000  , \"τC\"-> 0.000000000000  , \"κ0\"-> 0.000000000000  , \"mm1\"-> 0.000000000000  , \"mm2\"-> 0.000000000000  , \"mm3\"-> 0.000000000000  , \"T\"->  0.157000000000  , \"B\"-> 12.000000000000  , \"θ\"-> 45.000000000000  |>   , \r80126 ->   <| \"ζ\"->  0.000000000000  , \"τ1\"-> 0.000000000000  , \"τS\"-> 0.000000000000  , \"τN\"-> 0.000000000000  , \"τC\"-> 0.000000000000  , \"κ0\"-> 0.000000000000  , \"mm1\"-> 0.000000000000  , \"mm2\"-> 0.000000000000  , \"mm3\"-> 0.000000000000  , \"T\"->  0.120000000000  , \"B\"-> 12.000000000000  , \"θ\"-> 45.000000000000  |>   , \r80127 ->   <| \"ζ\"->  0.000000000000  , \"τ1\"-> 0.000000000000  , \"τS\"-> 0.000000000000  , \"τN\"-> 0.000000000000  , \"τC\"-> 0.000000000000  , \"κ0\"-> 0.000000000000  , \"mm1\"-> 0.000000000000  , \"mm2\"-> 0.000000000000  , \"mm3\"-> 0.000000000000  , \"T\"->  0.170000000000  , \"B\"-> 12.000000000000  , \"θ\"-> 45.000000000000  |>   , \r80128 ->   <| \"ζ\"->  0.000000000000  , \"τ1\"-> 0.000000000000  , \"τS\"-> 0.000000000000  , \"τN\"-> 0.000000000000  , \"τC\"-> 0.000000000000  , \"κ0\"-> 0.000000000000  , \"mm1\"-> 0.000000000000  , \"mm2\"-> 0.000000000000  , \"mm3\"-> 0.000000000000  , \"T\"->  0.200000000000  , \"B\"-> 12.000000000000  , \"θ\"-> 45.000000000000  |>   , \r80129 ->   <| \"ζ\"->  0.000000000000  , \"τ1\"-> 0.000000000000  , \"τS\"-> 0.000000000000  , \"τN\"-> 0.000000000000  , \"τC\"-> 0.000000000000  , \"κ0\"-> 0.000000000000  , \"mm1\"-> 0.000000000000  , \"mm2\"-> 0.000000000000  , \"mm3\"-> 0.000000000000  , \"T\"->  0.255000000000  , \"B\"-> 12.000000000000  , \"θ\"-> 45.000000000000  |>   , \r80130 ->   <| \"ζ\"->  0.000000000000  , \"τ1\"-> 0.000000000000  , \"τS\"-> 0.000000000000  , \"τN\"-> 0.000000000000  , \"τC\"-> 0.000000000000  , \"κ0\"-> 0.000000000000  , \"mm1\"-> 0.000000000000  , \"mm2\"-> 0.000000000000  , \"mm3\"-> 0.000000000000  , \"T\"->  0.300000000000  , \"B\"-> 12.000000000000  , \"θ\"-> 45.000000000000  |>   , \r80131 ->   <| \"ζ\"->  0.000000000000  , \"τ1\"-> 0.000000000000  , \"τS\"-> 0.000000000000  , \"τN\"-> 0.000000000000  , \"τC\"-> 0.000000000000  , \"κ0\"-> 0.000000000000  , \"mm1\"-> 0.000000000000  , \"mm2\"-> 0.000000000000  , \"mm3\"-> 0.000000000000  , \"T\"->  0.360000000000  , \"B\"-> 12.000000000000  , \"θ\"-> 45.000000000000  |>   , \r80132 ->   <| \"ζ\"->  0.000000000000  , \"τ1\"-> 0.000000000000  , \"τS\"-> 0.000000000000  , \"τN\"-> 0.000000000000  , \"τC\"-> 0.000000000000  , \"κ0\"-> 0.000000000000  , \"mm1\"-> 0.000000000000  , \"mm2\"-> 0.000000000000  , \"mm3\"-> 0.000000000000  , \"T\"->  0.430000000000  , \"B\"-> 12.000000000000  , \"θ\"-> 45.000000000000  |>   , \r80133 ->   <| \"ζ\"->  0.000000000000  , \"τ1\"-> 0.000000000000  , \"τS\"-> 0.000000000000  , \"τN\"-> 0.000000000000  , \"τC\"-> 0.000000000000  , \"κ0\"-> 0.000000000000  , \"mm1\"-> 0.000000000000  , \"mm2\"-> 0.000000000000  , \"mm3\"-> 0.000000000000  , \"T\"->  0.530000000000  , \"B\"-> 12.000000000000  , \"θ\"-> 45.000000000000  |>   , \r80134 ->   <| \"ζ\"->  0.000000000000  , \"τ1\"-> 0.000000000000  , \"τS\"-> 0.000000000000  , \"τN\"-> 0.000000000000  , \"τC\"-> 0.000000000000  , \"κ0\"-> 0.000000000000  , \"mm1\"-> 0.000000000000  , \"mm2\"-> 0.000000000000  , \"mm3\"-> 0.000000000000  , \"T\"->  0.620000000000  , \"B\"-> 12.000000000000  , \"θ\"
